vi "Emballage affiche cmde non terminée.vi"(0 "Nbre de valve dans carton":i16=8, 3 "melange des lots possibles ?":bool=TRUE, 7 "Nombre de carton+1":i16=2, 11 "error in (no error)":errorcluster caption="entrée d'erreur (pas d'erreur)", 12 "N° cmde en cours":string="00000/00-00.00.00") -> (2 "DATA cmde":T1={"n°article FAS"="", "n° cmde FAS"="02302/08-01.07.01", "quantité cmde"="100", "ID LIG cmde"="225785", "n° cmde client"="120189 / 109644     ", "nom client"="Fluid Automat. Systems GmbH", "n° article client"="20869", "indice revision client"="03    ", "société de facturation"="FAS Medic SA                            ", "langue a utiliser"="ALL"}, 4 "Recommencer la commande OUT":bool, 6 "Pb lecture cmde":bool, 8 "Continuer l'emballage  OUT":bool=TRUE, 15 "error out":errorcluster caption="sortie d'erreur")   [LabVIEW 2020]
uses:
  Modules/FS/60_FS_Controles/60_FS_SetGet.ctl
panel:
  out "Nombre de carton complets":i16
  in  "Recommencer la commande":bool
  out "pièce(s)":i16
  out "Nombre de carton+1 :":i16
  in  "Continuer l'emballage":bool
  # "Commande n°\n\nnon terminée !"
  # "Nombre de cartons emballés :"
  # "Vous avez \n dans le carton n°"
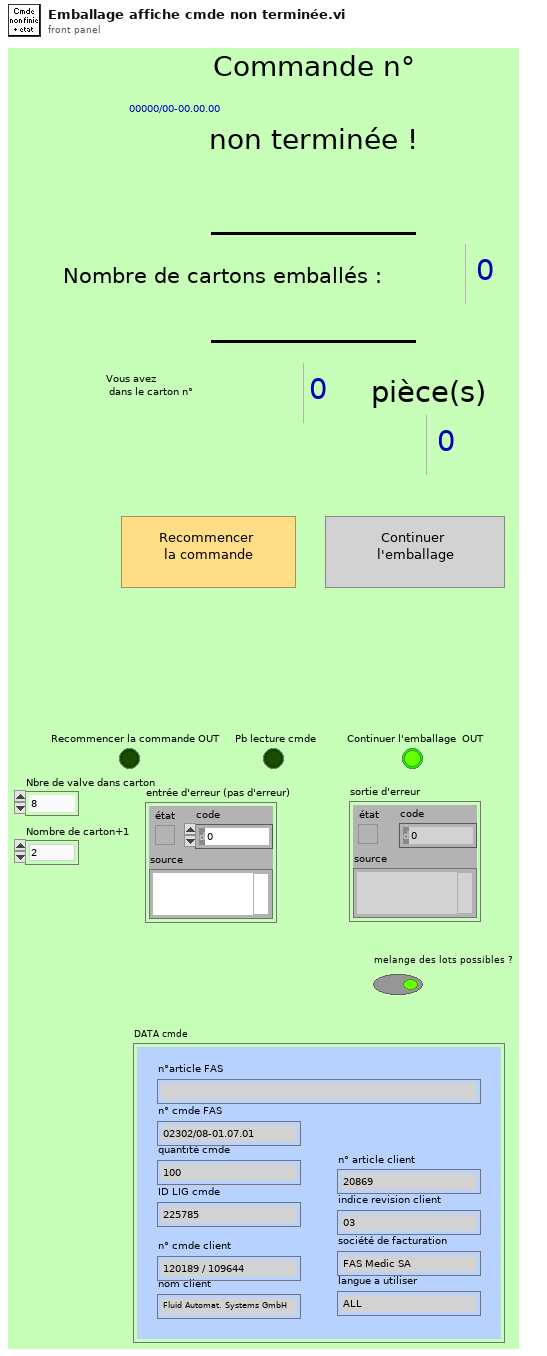
[diagram p1: front panel]
types:
  T1 = typedef "DATA commande.ctl" = cluster{"n°article FAS":string, "n° cmde FAS":string, "quantité cmde":string, "ID LIG cmde":string, "n° cmde client":string, "nom client":string, "n° article client":string, "indice revision client":string, "société de facturation":string, "langue a utiliser":string}
  T2 = enum8{"Enabled", "Disabled", "Disabled and Grayed Out"}
  T3 = typedef "60_FS_SetGet.ctl" = enum16{"set", "get"}
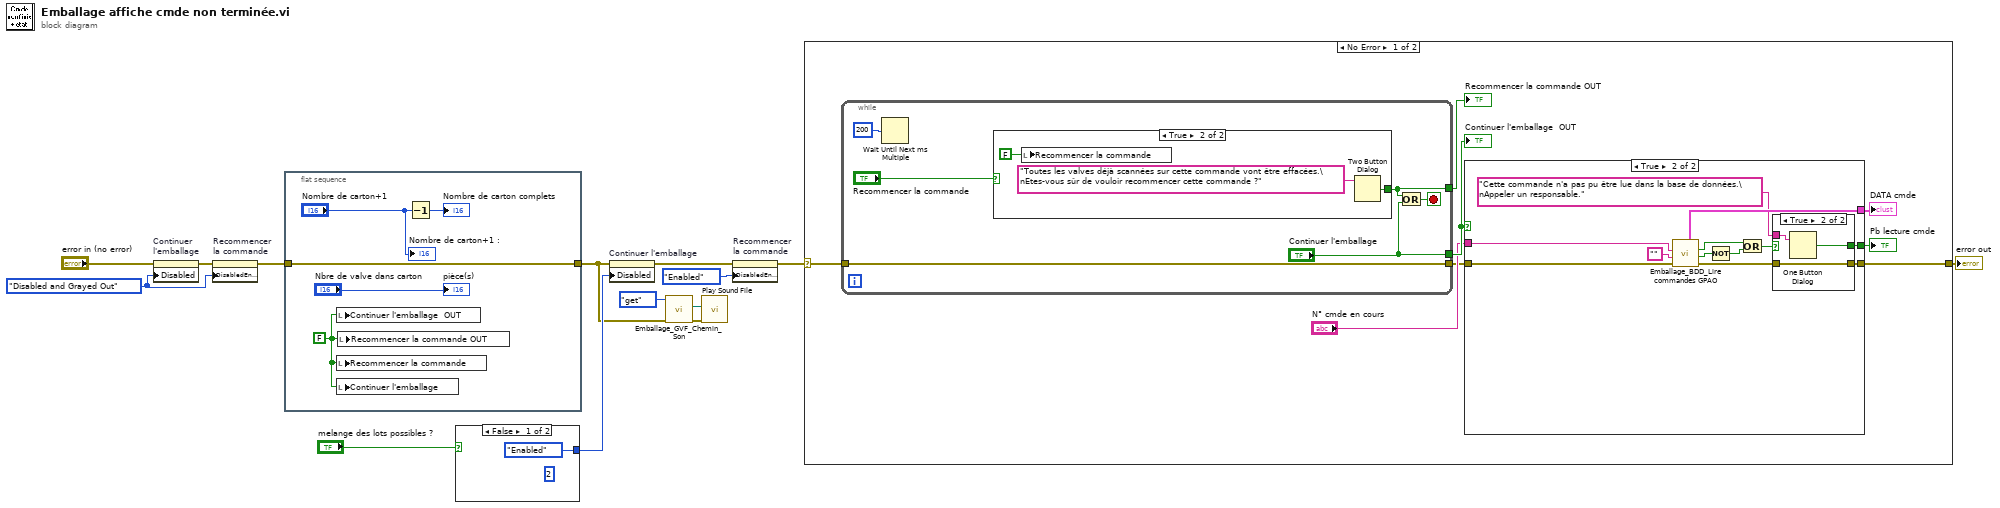
[diagram p0: block diagram]
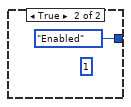
[diagram p2: hidden frame]
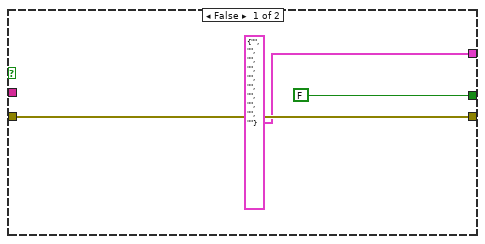
[diagram p3: hidden frame]
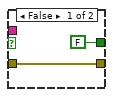
[diagram p4: hidden frame]
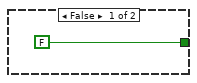
[diagram p5: hidden frame]
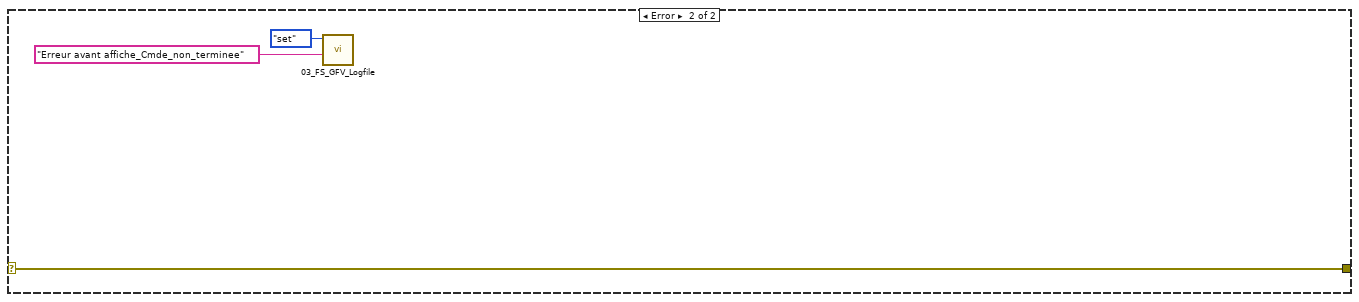
[diagram p6: hidden frame]
diagram:
  w3 = T2."Disabled and Grayed Out" ("Désactivé")
  n1 = property on="Continuer \nl'emballage" class="Bool (strict)"(error in="error in (no error)", "Disabled"=w3) -> (error out=w4:errorcluster)  [unwired: 1 in, 1 out]
  n2 = property on="Recommencer \nla commande" class="Bool (strict)"(error in=w4, "DisabledEnum"=w3) -> (error out=w1:errorcluster)  [unwired: 1 in, 1 out]
  n3 = flat-sequence {
    tunnel: [w15] -> w8
    tunnel: w1 -> [w15]
    frame #0 {
      w16 = FALSE
      n4 = local write "Continuer l'emballage  OUT"(w16) -> ()
      n5 = local write "Recommencer la commande"(w16) -> ()
      n6 = local write "Continuer l'emballage"(w16) -> ()
      n7 = local write "Recommencer la commande OUT"(w16) -> ()
      n8 = Decrement(x="Nombre de carton+1") -> (x-1=→"Nombre de carton complets":i16)
      "Nombre de carton+1 :" <- "Nombre de carton+1"
      "pièce(s)" <- "Nbre de valve dans carton"
    }
  }
  n9 = case shown="False" "melange des lots possibles ?" {
    tunnel: [T2."Enabled" ("Désactivé") T2."Enabled" ("Désactivé")] -> w12
    frame False {
      (unwired) 2
    }
    frame True {
      (unwired) 1
    }
  }
  n10 = property on="Continuer l'emballage" class="Bool (strict)"(error in=w8, "Disabled"=w12) -> (error out=w7:errorcluster)  [unwired: 1 in, 1 out]
  n11 = call "Emballage_GVF_Chemin_Son.vi"("entrée d'erreur (pas d'erreur)"=w8, "Énum"=enum16{"get", "set"}."get") -> ("sortie d'erreur"=w11:errorcluster, "Chemin Utopia - Question.WAV"=w10:path)  [unwired: 5 in, 3 out]
  n12 = call <vilib>:"Play Sound File.vi"("error in (no error)"=w11, "path"=w10) -> ()  [unwired: 8 in, 2 out]
  n13 = property on="Recommencer \nla commande" class="Bool (strict)"(error in=w7, "DisabledEnum"=T2."Enabled" ("Désactivé")) -> (error out=w6:errorcluster)  [unwired: 1 in, 1 out]
  n14 = case shown="No Error" w6 {
    selector: w6 -> [w23 w62]
    tunnel: [w28 w62] -> w14
    frame No Error {
      n15 = while {
        tunnel: ["Continuer l'emballage"] -> w29
        tunnel: [w51] -> w24
        tunnel: [w52] -> w22
        tunnel: w23 -> [w52]
        stop <- w54 stop-if-true
        n16 = Wait Until Next ms Multiple(millisecond multiple=200) -> ()  [unwired: 1 out]
        n17 = case shown="True" "Recommencer la commande" {
          tunnel: [FALSE ("T button?") w58] -> w51
          frame False {
          }
          frame True {
            n18 = local write "Recommencer la commande"(FALSE ("Recommencer la commande")) -> ()
            n19 = Two Button Dialog(message="Toutes les valves déjà scannées sur cette commande vont être effacées.\nEtes-vous sûr de vouloir recommencer cette commande ?") -> (T button?=w58:bool)  [unwired: 2 in]
          }
        }
        n20 = Or(x=w51, y="Continuer l'emballage") -> (x .or. y?=w54:bool)
      }
      "Continuer l'emballage  OUT" <- w29
      "Recommencer la commande OUT" <- w24
      n21 = case shown="True" w29 {
        tunnel: w22 -> [w32 w42]
        tunnel: [w32 w33] -> w28
        tunnel: [T1 {"n°article FAS"="", "n° cmde FAS"="", "quantité cmde"="", "ID LIG cmde"="", "n° cmde client"="", "nom client"="", "n° article client"="", "indice revision client"="", "société de facturation"="", "langue a utiliser"=""} ("DATA cmde") w38] -> w27
        tunnel: "N° cmde en cours" -> [_ w41]
        tunnel: [FALSE ("OK") w36] -> w25
        frame False {
        }
        frame True {
          n22 = call "Emballage_BDD_Lire  commandes GPAO.vi"("error in"=w42, "article"="", "Numéro commande"=w41) -> ("error out"=w34:errorcluster, "existe ?"=w39:bool, "Erreur de\n comunication"=w40:bool, "DATA cmde"=w38:T1)  [unwired: 3 in, 2 out]
          n23 = Not(x=w39) -> (.not. x?=w44:bool)
          n24 = Or(x=w40, y=w44) -> (x .or. y?=w35:bool)
          n25 = case shown="True" w35 {
            tunnel: "Cette commande n'a pas pu être lue dans la base de données.\nAppeler un responsable." ("Message") -> [_ w49]
            tunnel: [FALSE ("true") w48] -> w36
            tunnel: w34 -> [w45 w47]
            tunnel: [w45 w47] -> w33
            frame False {
            }
            frame True {
              n26 = One Button Dialog(message=w49) -> (true=w48:bool)  [unwired: 1 in]
            }
          }
        }
      }
      "Pb lecture cmde" <- w25
      "DATA cmde" <- w27
    }
    frame Error {
      n27 = call "03_FS_GFV_Logfile.vi"("Chaîne"="Erreur avant affiche_Cmde_non_terminee", "States"=60_FS_SetGet."set") -> ()  [unwired: 8 in, 2 out]
    }
  }
  "error out" <- w14
